vi "DBManip-SortDateColumn.vi"(5 "Sorting Order":enum16{"ascending", "descending"}(ring), 7 "disabled index (col)":i32=3, 8 "error in":errorcluster, 11 "DB Table Data":string[][](array[string])=[["1", "tej", "2/28/13", "3/15/2013", "123456987987", "This is a dummy test", "50", "dummy instructions", "unassigned", "2/28/13", "1234556"], ["2", "tej", "2/28/13", "1/25/2013", "123456987987", "This is a dummy test", "50", "dummy instructions", "unassigned", "2/28/13", "1234556"], ["4", "tej", "2/28/13", "3/25/2013", "123456987987", "This is a dummy test", "50", "dummy instructions", "unassigned", "2/28/13", "1234556"], ["6", "tej", "2/28/13", "12/05/2012", "123456987987", "This is a dummy test", "50", "dummy instructions", "unassigned", "2/28/13", "1234556"]]) -> (0 "error out":errorcluster, 3 "Sorted Data by Date":string[][](array[string]))   [LabVIEW 2013]
uses:
  <userlib>/_OpenG.lib/array/array.llb/Sort 1D Array (I32)__ogtk.vi
  <userlib>/_OpenG.lib/array/array.llb/Reorder 2D Array2 (String)__ogtk.vi
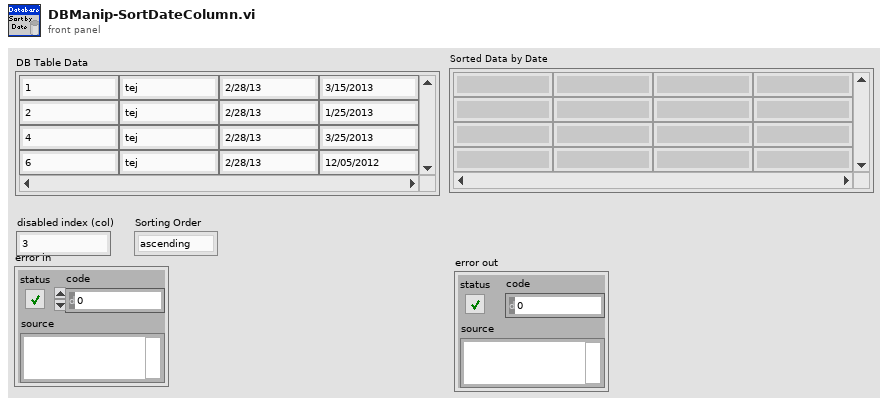
[diagram p1: front panel]
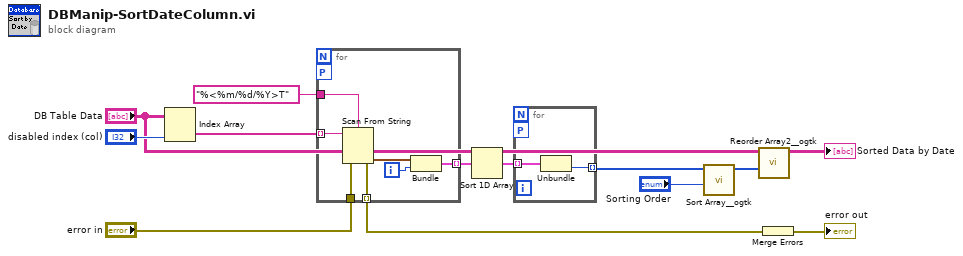
[diagram p0: block diagram]
diagram:
  n1 = Index Array(array="DB Table Data", index (col)="disabled index (col)") -> (element=w13:string[])  [unwired: 1 in]
  n2 = for {
    tunnel: "%<%m/%d/%Y>T" ("format string") -> [w20]
    tunnel: w13 -> [w19] mode=indexing
    tunnel: [w16] -> w7 mode=indexing
    tunnel: "error in" -> [w15]
    tunnel: [w14] -> w5 mode=indexing
    workers-P: _ -> [_]
    i -> [w17]
    n3 = Scan From String(format string=w20, input string=w19, error in=w15) -> (error out=w14:errorcluster, output 1=w18:timestamp)  [unwired: 2 in, 2 out]
    n4 = Bundle(w18, w17) -> (w16:cluster{timestamp, i32})  [unwired: 1 in]
  }
  n5 = Sort 1D Array(array=w7) -> (sorted array=w8:cluster{timestamp, i32}[])
  n6 = for {
    tunnel: w8 -> [w22] mode=indexing
    tunnel: [w21] -> w3 mode=indexing
    workers-P: _ -> [_]
    n7 = Unbundle(w22) -> (w21:i32)  [unwired: 1 out]
  }
  n8 = call-poly <userlib>:"Sort Array__ogtk.vi"("Order"="Sorting Order", "Array in"=w3) -> ("Sorted Array out"=w1:i32[])  [unwired: 8 in, 1 out]
  n9 = call-poly <userlib>:"Reorder Array2__ogtk.vi"("indices"=w1, "array"="DB Table Data") -> ("reordered array"=→"Sorted Data by Date":string[][])  [unwired: 9 in]
  n10 = Merge Errors(w5) -> (→"error out":errorcluster)
